vi "1.arithmatics.vi"() -> ()   [LabVIEW 2010]
panel:
  in  "Slide 4":dbl(slide) scale=0.0..10.0
  in  "Slide 3":dbl(slide) scale=0.0..10.0
  out "Tank":dbl(slide) scale=0.0..10.0
  in  "Slide 2":dbl(slide) scale=0.0..10.0
  in  "Slide":dbl(slide) scale=0.0..10.0
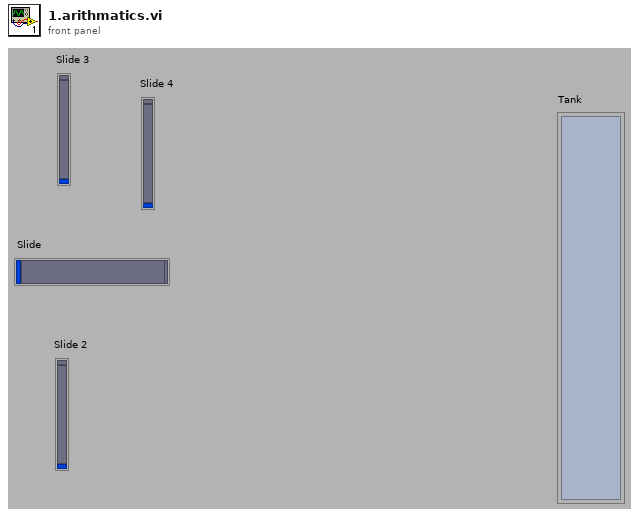
[diagram p1: front panel]
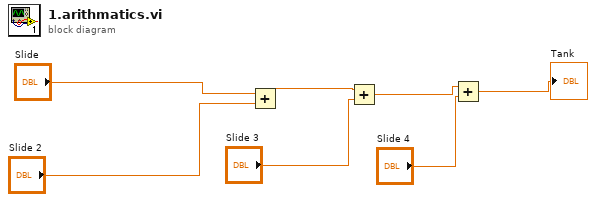
[diagram p0: block diagram]
diagram:
  n1 = Add(x="Slide", y="Slide 2") -> (x+y=w5:dbl)
  n2 = Add(x=w5, y="Slide 3") -> (x+y=w4:dbl)
  n3 = Add(x=w4, y="Slide 4") -> (x+y=→"Tank":dbl)
